vi "testScriptCompiler.vi"(10 "Path":path) -> ()   [LabVIEW 2011, in "run.lvlib"]
uses:
  run.lvlib
  Tools/DatabaseHelpers/DbConnection/DeviceDataBase/deviceDataBase.lvclass
  Channels/Digital/DigitalOutput.lvclass
  Channels/VoltOutput/AnalogOutput.lvclass
  Channels/DDSOutput/Generic/DDSOutput.lvclass
  Tools/Filing/FileNeologist/FileNeologist.lvclass
  Tools/DataMappers/DeviceData/DeviceData.lvclass
  Tools/DataMappers/DeviceData/DoDeviceData/DoDeviceData.lvclass
  Tools/DataMappers/DeviceData/AoDeviceData/AoDeviceData.lvclass
  Tools/DataMappers/DeviceData/RfOutputData/RfOutputData.lvclass
  Tools/SettingsProcessors/ScriptListCompiler/ScriptListCompiler.lvclass
  Tools/DatabaseHelpers/Database Objects/DeviceArray/DeviceArray.lvclass
  Tools/DatabaseHelpers/Database Objects/device/device.lvclass
  Tools/Scripting/ScriptingEvent/ScriptEventList/ScriptEventList.lvclass
  Tools/Filing.lvlib
panel:
  out "times":dbl[](array[numeric])
  out "Number of triggers":i32
  in  "channel_index":i32=9
  out "database out":refnum<class "deviceDataBase.lvclass">
  out "DB":dbl format="%_9g"
  out "error out":errorcluster
  out "rfDataArray":cluster{dbl[][]}[](array[cluster])
  out "rf physicalChannels":string[](array[string])
  in  "Channel Nr":i32
  out "timingDo":dbl
  out "timingAO":dbl
  out "compiler":dbl
  out "eventStringArray":string[][][](array[string])
  out "digital Data":T1 {"Timestamps ms" format="%_11g"}
  out "Timing 2":T2
  out "analog data":dbl[][](array[numeric])
  out "Ranges":dbl[](array[numeric])
  out "Physical Channels 2":string
  out "Digital":string
  out "Routings":cluster{"Master Clock Route":string[]}
  out "Timing":T3
  out "Physical Channels":string
  out "AO channel":string
  out "timing":dbl
  # "time does not include\nopen database\ntime"
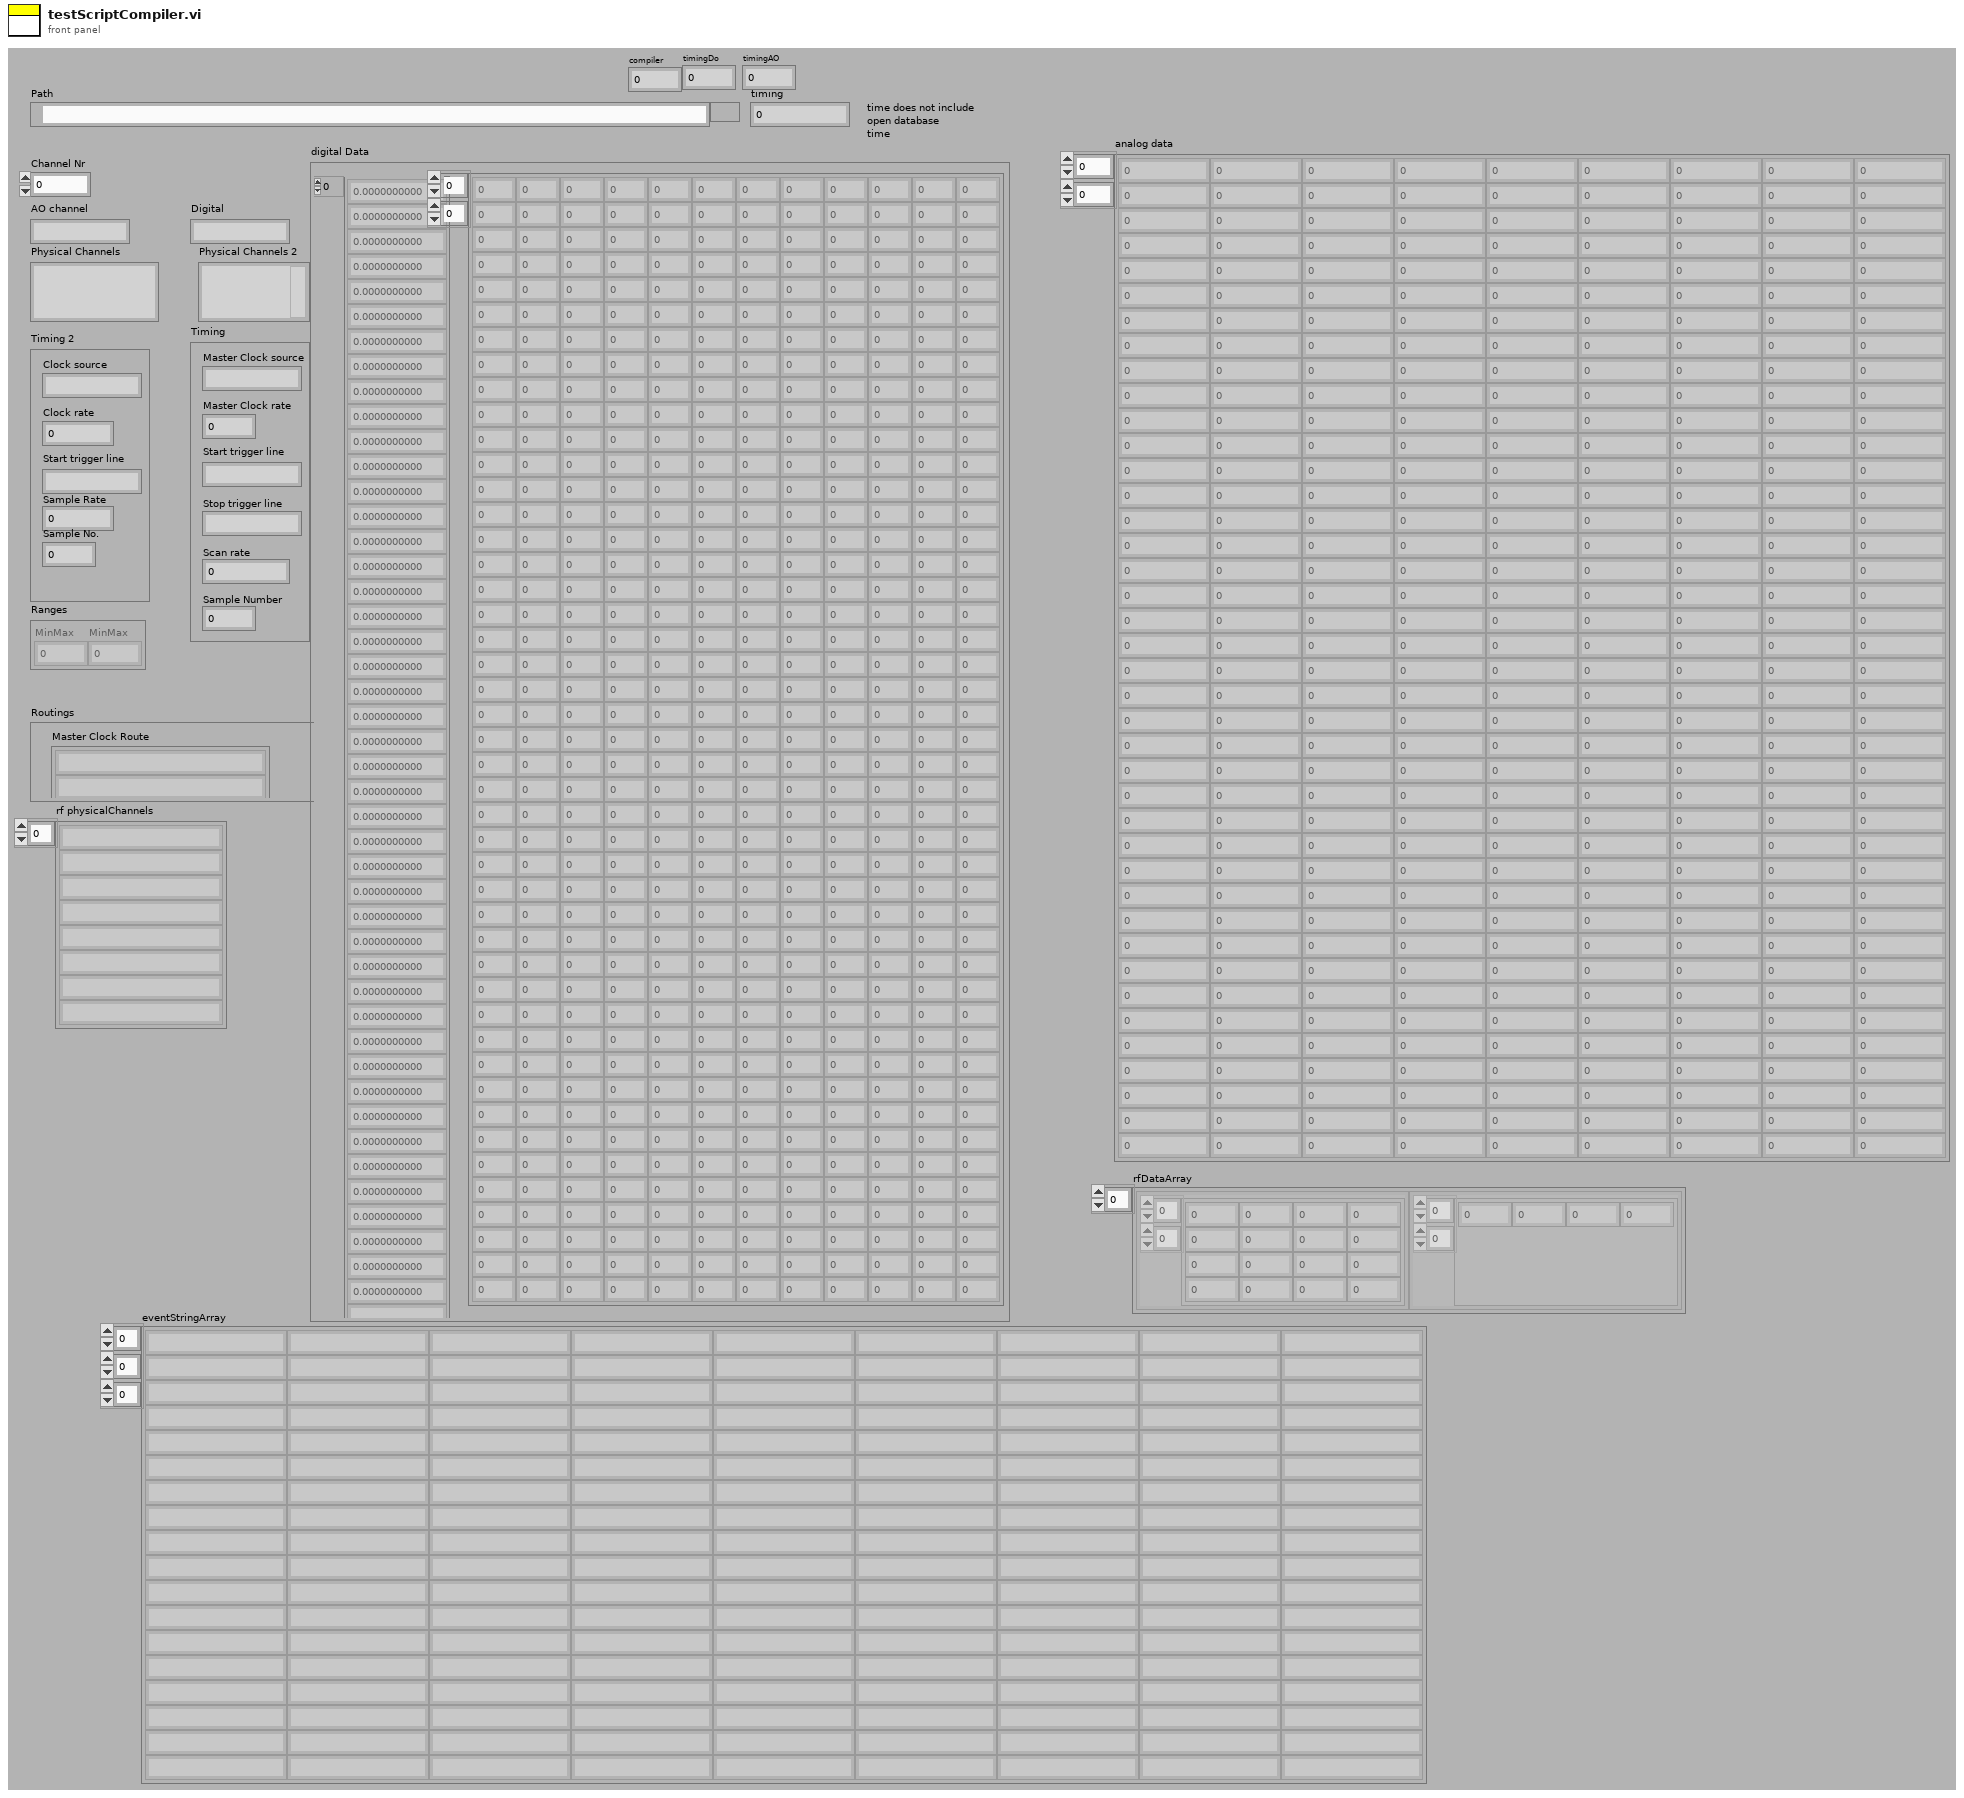
[diagram p1: front panel]
types:
  T1 = cluster{"Timestamps ms":dbl[], "DataPerChannel":dbl[][]}
  T2 = cluster{"Clock source":string, "Clock rate":dbl, "Start trigger line":string, "Sample Rate":dbl, "Sample No.":dbl}
  T3 = cluster{"Master Clock source":string, "Master Clock rate":dbl, "Start trigger line":string, "Scan rate":dbl, "Stop trigger line":string, "Sample Number":dbl}
  T4 = enum16{"digitalOutput", "digitalInput", "analogOutput", "analogInput", "rfOutput", "ethernetSupply"}
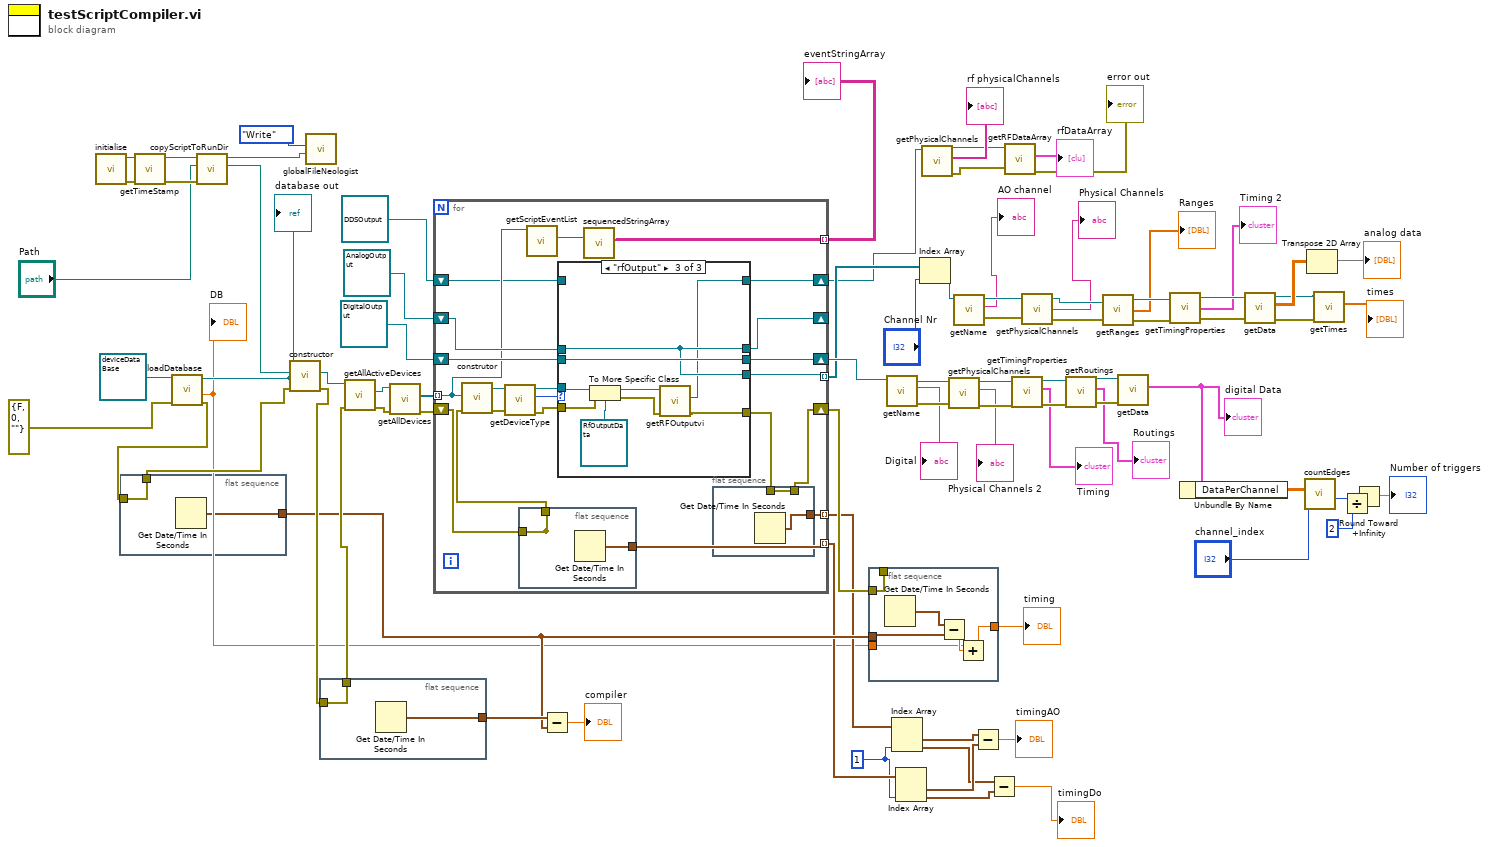
[diagram p0: block diagram]
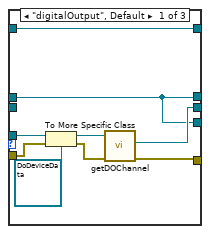
[diagram p2: hidden frame]
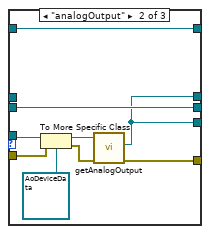
[diagram p3: hidden frame]
diagram:
  w55 = 1
  n1 = call "initialise.vi"() -> ("error out"=w79:errorcluster, "FileNeologist out"=w78:refnum<class "FileNeologist.lvclass">)  [unwired: 10 in]
  n2 = flat-sequence {
    tunnel: [w87] -> w63
    tunnel: w22 -> [w86]
    tunnel: [w86] -> w21
    frame #0 {
      n3 = Get Date/Time In Seconds() -> (seconds since 1Jan1904=w87:timestamp)
    }
  }
  n4 = call "getTimeStamp.vi"("error in (no error)"=w79, "FileNeologist in"=w78) -> ("error out"=w77:errorcluster, "FileNeologist out"=w76:refnum<class "FileNeologist.lvclass">)  [unwired: 7 in, 1 out]
  n5 = call "loadDatabase.vi"("error in (no error)"=errorcluster {"status"=FALSE, "code"=0, "source"=""}, "deviceDataBase in"=refnum<class "deviceDataBase.lvclass"> refnum) -> ("error out"=w22:errorcluster, "total"=w1:dbl, "deviceDataBase out"=w13:refnum<class "deviceDataBase.lvclass">)  [unwired: 7 in]
  "DB" <- w1
  "database out" <- w13
  n6 = call-dynamic "copyScriptToRunDir.vi"("error in (no error)"=w77, "Path in"="Path", "FileNeologist in"=w76) -> ("Path out"=w75:path, "FileNeologist out"=w67:refnum<class "FileNeologist.lvclass">)  [unwired: 6 in, 1 out]
  n7 = call "constructor.vi"("error in (no error)"=w21, "deviceDataBase"=w13, "Path"=w75) -> ("error out"=w66:errorcluster, "DeviceArray"=w74:refnum<class "DeviceArray.lvclass">)  [unwired: 5 in, 2 out]
  n8 = call "globalFileNeologist.vi"("FileNeologist in"=w67, "Action"=enum16{"Write", "Read"}."Write") -> ()  [unwired: 9 in, 1 out]
  n9 = flat-sequence {
    tunnel: [w89] -> w64
    tunnel: w66 -> [w88]
    tunnel: [w88] -> w65
    frame #0 {
      n10 = Get Date/Time In Seconds() -> (seconds since 1Jan1904=w89:timestamp)
    }
  }
  n11 = call "getAllActiveDevices.vi"("error in (no error)"=w65, "DeviceArray in"=w74) -> ("error out"=w73:errorcluster, "DeviceArray"=w72:refnum<class "DeviceArray.lvclass">)  [unwired: 7 in, 1 out]
  n12 = call "getAllDevices.vi"("error in (no error)"=w73, "DeviceArray.lvclass in"=w72) -> ("error out"=w70:errorcluster, "deviceArray"=w71:refnum<class "device.lvclass">[])  [unwired: 7 in, 1 out]
  n13 = for {
    shift-right: [w94] -> w81
    shift-left: w70 -> [w98]
    shift-right: [w106] -> w80
    shift-left: refnum<class "DigitalOutput.lvclass"> refnum ("DigitalOutput") -> [w105]
    shift-right: [w104] -> _
    shift-left: refnum<class "AnalogOutput.lvclass"> refnum ("aOChannel") -> [w103]
    tunnel: w71 -> [w100] mode=indexing
    tunnel: [w99] -> w69 mode=indexing
    tunnel: [w96] -> w60 mode=indexing
    tunnel: [w93] -> w61 mode=indexing
    tunnel: [w92] -> w26 mode=indexing
    shift-right: [w90] -> w19
    shift-left: refnum<class "DDSOutput.lvclass"> refnum ("Hardware:Channels.lvlib:DDSOutput.lvclass") -> [w91]
    n14 = call "construtor.vi"("error in (no error)"=w97, "device"=w100) -> ("error out"=w110:errorcluster, "DeviceData out"=w109:refnum<class "DeviceData.lvclass">)  [unwired: 8 in]
    n15 = call-dynamic "getDeviceType.vi"("error in (no error)"=w110, "DeviceData in"=w109) -> ("error out"=w102:errorcluster, "type"=w108:T4, "DeviceData out"=w107:refnum<class "DeviceData.lvclass">)  [unwired: 7 in]
    n16 = flat-sequence {
      tunnel: [w114] -> _
      tunnel: [w114] -> w97
      tunnel: w98 -> [w114]
      tunnel: [w113] -> w96
      frame #0 {
        n17 = Get Date/Time In Seconds() -> (seconds since 1Jan1904=w113:timestamp)
      }
    }
    n18 = call "getScriptEventList.vi"("device.lvclass in"=w100) -> ("ScriptEventList"=w101:refnum<class "ScriptEventList.lvclass">)  [unwired: 8 in, 2 out]
    n19 = case shown="\"rfOutput\"" w108 {
      tunnel: w107 -> [w123 w131 w141]
      tunnel: [w120 w128 w140] -> w106
      tunnel: w105 -> [_ w128 w140]
      tunnel: [w116 w125 w134] -> w104
      tunnel: w103 -> [w116 _ w134]
      tunnel: w102 -> [w119 w127 w139]
      tunnel: [w117 w126 w135] -> w95
      tunnel: [w116 w125 w134] -> w92
      tunnel: w91 -> [w115 w124 _]
      tunnel: [w115 w124 w133] -> w90
      frame "digitalOutput", Default {
        n20 = To More Specific Class(target class=refnum<class "DoDeviceData.lvclass"> refnum ("DoDeviceData.lvclass in"), reference=w123, error in=w119) -> (specific class reference=w121:refnum<class "DoDeviceData.lvclass">, error out=w118:errorcluster)
        n21 = call "getDOChannel.vi"("error in (no error)"=w118, "DoDeviceData.lvclass in"=w121) -> ("error out"=w117:errorcluster, "DigitalOutput"=w120:refnum<class "DigitalOutput.lvclass">)  [unwired: 7 in, 1 out]
      }
      frame "analogOutput" {
        n22 = To More Specific Class(target class=refnum<class "AoDeviceData.lvclass"> refnum ("AoDeviceData.lvclass in"), reference=w131, error in=w127) -> (specific class reference=w129:refnum<class "AoDeviceData.lvclass">, error out=w132:errorcluster)
        n23 = call "getAnalogOutput.vi"("error in (no error)"=w132, "AoDeviceData.lvclass in"=w129) -> ("error out"=w126:errorcluster, "aOChannel"=w125:refnum<class "AnalogOutput.lvclass">)  [unwired: 7 in, 1 out]
      }
      frame "rfOutput" {
        n24 = To More Specific Class(target class=refnum<class "RfOutputData.lvclass"> refnum ("DataMappers.lvlib:RfOutputData.lvclass"), reference=w141, error in=w139) -> (specific class reference=w137:refnum<class "RfOutputData.lvclass">, error out=w136:errorcluster)
        n25 = call-dynamic "getRFOutputvi.vi"("error in (no error)"=w136, "RfOutputData in"=w137) -> ("error out"=w135:errorcluster, "DDSOutput"=w133:refnum<class "DDSOutput.lvclass">)  [unwired: 7 in, 1 out]
      }
    }
    n26 = call "sequencedStringArray.vi"("ScriptEventList in"=w101) -> ("eventStringArray"=w99:string[][])  [unwired: 8 in, 2 out]
    n27 = flat-sequence {
      tunnel: [w112] -> w93
      tunnel: w95 -> [w111]
      tunnel: [w111] -> _
      tunnel: [w111] -> w94
      frame #0 {
        n28 = Get Date/Time In Seconds() -> (seconds since 1Jan1904=w112:timestamp)
      }
    }
  }
  "eventStringArray" <- w69
  n29 = Subtract(x=w64, y=w63) -> (x-y=→"compiler":dbl)
  n30 = flat-sequence {
    tunnel: w63 -> [w146]
    tunnel: [w144] -> w84
    tunnel: w81 -> [w145]
    tunnel: [w145] -> _
    tunnel: w1 -> [w142]
    frame #0 {
      n31 = Get Date/Time In Seconds() -> (seconds since 1Jan1904=w147:timestamp)
      n32 = Subtract(x=w147, y=w146) -> (x-y=w143:dbl)
      n33 = Add(x=w142, y=w143) -> (x+y=w144:dbl)
    }
  }
  n34 = call-dynamic "getName.vi"("DigitalOutput.lvclass in"=w80) -> ("error out"=w38:errorcluster, "name"=→"Digital":string, "DigitalOutput.lvclass out"=w39:refnum<class "DigitalOutput.lvclass">)  [unwired: 8 in]
  n35 = Index Array(array=w61, index #2=w55) -> (element #1=w59:timestamp, element #2=w57:timestamp)  [unwired: 1 in]
  n36 = Index Array(array=w60, index #2=w55) -> (element #1=w58:timestamp, element #2=w56:timestamp)  [unwired: 1 in]
  n37 = Index Array(array=w26, index="Channel Nr") -> (element=w25:refnum<class "AnalogOutput.lvclass">)
  n38 = call "getPhysicalChannels.vi"("DDSOutput in"=w19) -> ("error out"=w16:errorcluster, "physicalChannels"=→"rf physicalChannels":string[], "DDSOutput out"=w17:refnum<class "DDSOutput.lvclass">)  [unwired: 8 in]
  n39 = call-dynamic "getPhysicalChannels.vi"("error in (no error)"=w38, "DigitalOutput.lvclass in"=w39) -> ("error out"=w36:errorcluster, "Physical Channels"=→"Physical Channels 2":string, "DigitalOutput.lvclass out"=w37:refnum<class "DigitalOutput.lvclass">)  [unwired: 7 in]
  n40 = call "getName.vi"("AnalogOutput.lvclass in"=w25) -> ("error out"=w52:errorcluster, "name"=→"AO channel":string, "AnalogOutput.lvclass out"=w48:refnum<class "AnalogOutput.lvclass">)  [unwired: 8 in]
  n41 = Subtract(x=w59, y=w58) -> (x-y=→"timingAO":dbl)
  n42 = Subtract(x=w57, y=w56) -> (x-y=→"timingDo":dbl)
  n43 = call "getRFDataArray.vi"("error in (no error)"=w16, "DDSOutput in"=w17) -> ("error out"=→"error out":errorcluster, "rfDataArray"=→"rfDataArray":cluster{dbl[][]}[])  [unwired: 7 in, 1 out]
  n44 = call-dynamic "getTimingProperties.vi"("error in (no error)"=w36, "DigitalOutput.lvclass in"=w37) -> ("error out"=w34:errorcluster, "Timing"=→"Timing":T3, "DigitalOutput.lvclass out"=w35:refnum<class "DigitalOutput.lvclass">)  [unwired: 7 in]
  n45 = call-dynamic "getPhysicalChannels.vi"("AnalogOutput.lvclass in"=w48, "error in (no error)"=w52) -> ("AnalogOutput.lvclass out"=w47:refnum<class "AnalogOutput.lvclass">, "Physical Channels"=→"Physical Channels":string, "error out"=w51:errorcluster)
  n46 = call-dynamic "getRoutings.vi"("error in (no error)"=w34, "DigitalOutput.lvclass in"=w35) -> ("error out"=w32:errorcluster, "Routings"=→"Routings":cluster{"Master Clock Route":string[]}, "DigitalOutput.lvclass out"=w33:refnum<class "DigitalOutput.lvclass">)  [unwired: 7 in]
  n47 = call "getRanges.vi"("AnalogOutput.lvclass in"=w47, "error in (no error)"=w51) -> ("AnalogOutput.lvclass out"=w46:refnum<class "AnalogOutput.lvclass">, "Ranges"=→"Ranges":dbl[], "error out"=w50:errorcluster)
  n48 = call-dynamic "getData.vi"("error in (no error)"=w32, "DigitalOutput.lvclass in"=w33) -> ("Data"=w11:T1)  [unwired: 7 in, 2 out]
  "digital Data" <- w11
  n49 = call "getTimingProperties.vi"("AnalogOutput.lvclass in"=w46, "error in (no error)"=w50) -> ("AnalogOutput.lvclass out"=w45:refnum<class "AnalogOutput.lvclass">, "Timing"=→"Timing 2":T2, "error out"=w49:errorcluster)
  n50 = Unbundle By Name(w11) -> ("DataPerChannel"=w10:dbl[][])
  n51 = call "getData.vi"("error in (no error)"=w49, "AnalogOutput.lvclass in"=w45) -> ("error out"=w3:errorcluster, "Data"=w40:dbl[][], "AnalogOutput.lvclass out"=w4:refnum<class "AnalogOutput.lvclass">)  [unwired: 7 in]
  n52 = call "countEdges.vi"("channel_index"="channel_index", "DataPerChannel"=w10) -> ("Number of Changes"=w8:i32)  [unwired: 8 in, 1 out]
  n53 = Transpose 2D Array(2D array=w40) -> (transposed array=→"analog data":dbl[][])
  n54 = call "getTimes.vi"("error in (no error)"=w3, "AnalogOutput in"=w4) -> ("times"=→"times":dbl[])  [unwired: 7 in, 2 out]
  n55 = Divide(x=w8, y=2) -> (x/y=w7:dbl)
  n56 = Round Toward +Infinity(x=w7) -> (ceil(x): smallest int >= x=→"Number of triggers":dbl)
  "timing" <- w84
